vi "FTW-dotNET-MySQL-ExecuteScript.vi"(0 "DB Connection":refnum<k24>, 5 "SQL Script":string, 11 "error in":errorcluster) -> (4 "DB Connection":refnum<k24>, 6 "Elapsed Time":dbl format="%.4psec", 15 "error out":errorcluster)   [LabVIEW 2015]
uses:
  MySql.Data
panel:
  # "Inputs"
  # "Outputs"
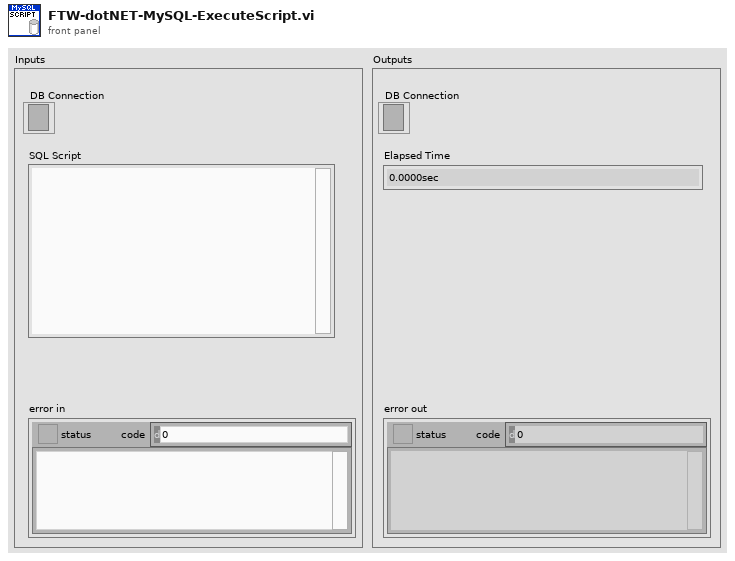
[diagram p1: front panel]
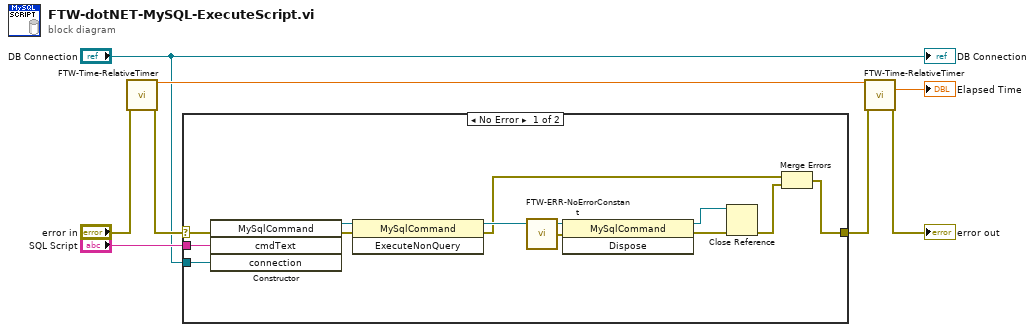
[diagram p0: block diagram]
diagram:
  n1 = call "FTW-Time-RelativeTimer.vi"("error in"="error in") -> ("Current Timer Value"=w5:dbl, "error out"=w6:errorcluster)  [unwired: 12 in, 1 out]
  n2 = case shown="No Error" w6 {
    selector: w6 -> [w11 w21]
    tunnel: "SQL Script" -> [w12 _]
    tunnel: [w13 w21] -> w2
    tunnel: "DB Connection" -> [w9 _]
    frame No Error {
      n3 = constructor class="MySqlCommand"(error in=w11, "cmdText"=w12, "connection"=w9) -> (reference out=w20:refnum<k24>, error out=w19:errorcluster)  [unwired: 2 in, 3 out]
      n4 = invoke on="Invoke Node" class="MySqlCommand" method="ExecuteNonQuery"(reference=w20, error in=w19) -> (reference out=w15:refnum<k24>, error out=w10:errorcluster)  [unwired: 1 in, 1 out]
      n5 = call "FTW-ERR-NoErrorConstant.vi"() -> ("no error"=w16:errorcluster)
      n6 = invoke class="MySqlCommand" method="Dispose"(reference=w15, error in=w16) -> (reference out=w17:refnum<k24>, error out=w18:errorcluster)  [unwired: 1 in, 1 out]
      n7 = Close Reference(reference=w17, error in (no error)=w18) -> (error out=w14:errorcluster)
      n8 = Merge Errors(w10, w14) -> (w13:errorcluster)
    }
    frame Error {
    }
  }
  n9 = call "FTW-Time-RelativeTimer.vi"("Previous Timer Value"=w5, "error in"=w2) -> ("Elapsed Time"=→"Elapsed Time":dbl, "error out"=→"error out":errorcluster)  [unwired: 11 in, 1 out]
  "DB Connection" <- "DB Connection"
